vi "Prepare DCPower.vi"(8 "error in":errorcluster, 9 "Channel List in":string, 10 "Instrument Handle in":refnum<k15> caption="instrument handle", 11 "Measurement Configuration in":T1={"Resource Name"="", "Measure Trigger Source"="", "Run Until"=6.0, "Current Limit"=0.01, "Voltage Level"=0.01, "Current Limit Range"=0.0, "Voltage Level Range"=5.0, "Aperture Time"=0.01666, "Current Unit"="mA", "Delimited Text"=","} {"Aperture Time" format="%#_6ps"; "Voltage Level Range" format="%#_6pV"; "Current Limit Range" format="%#_6pA"; "Voltage Level" format="%#_6pV"; "Current Limit" format="%#_6pA"; "Run Until" min=1.0 step=1.0 format="%#_g Samples"}) -> (0 "error out":errorcluster, 1 "Channel List out":string, 2 "Instrument Handle out":refnum<k15>, 3 "Measurement Configuration out":T1 {"Aperture Time" format="%#_6ps"; "Voltage Level Range" format="%#_6pV"; "Current Limit Range" format="%#_6pA"; "Voltage Level" format="%#_6pV"; "Current Limit" format="%#_6pA"; "Run Until" min=1.0 step=1.0 format="%#_g Samples"})   [LabVIEW 2025, in "DCPower Single Meas Per Trigger.lvclass"]
uses:
  DCPower Single Meas Per Trigger.lvclass
  Measurement Configuration.ctl
  <instrlib>/niDCPower/nidcpower.llb/niDCPower Output Function.ctl
  <instrlib>/niDCPower/nidcpower.llb/niDCPower Auto Zero.ctl
  <instrlib>/niDCPower/nidcpower.llb/niDCPower Aperture Time Units.ctl
  DCPower Single Meas Per Trigger.lvclass/DCPower Single Meas Per Trigger.ctl
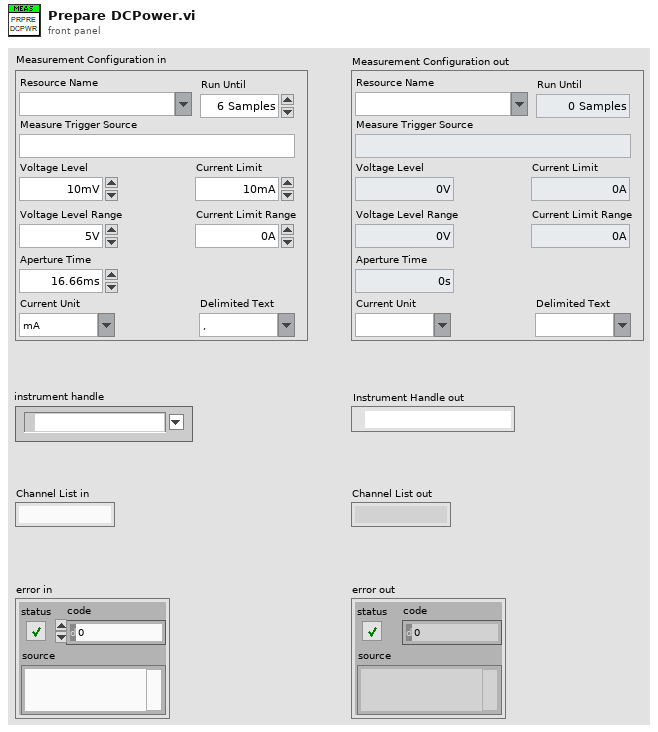
[diagram p1: front panel]
types:
  T1 = typedef "DCPower Single Meas Per Trigger.lvclass/Measurement Configuration.ctl" = cluster{"Resource Name":string, "Measure Trigger Source":string, "Run Until":dbl, "Current Limit":dbl, "Voltage Level":dbl, "Current Limit Range":dbl, "Voltage Level Range":dbl, "Aperture Time":dbl, "Current Unit":string, "Delimited Text":string}
  T2 = typedef "niDCPower Auto Zero.ctl" = i32
  T3 = typedef "niDCPower Output Function.ctl" = i32
  T4 = typedef "niDCPower Aperture Time Units.ctl" = i32
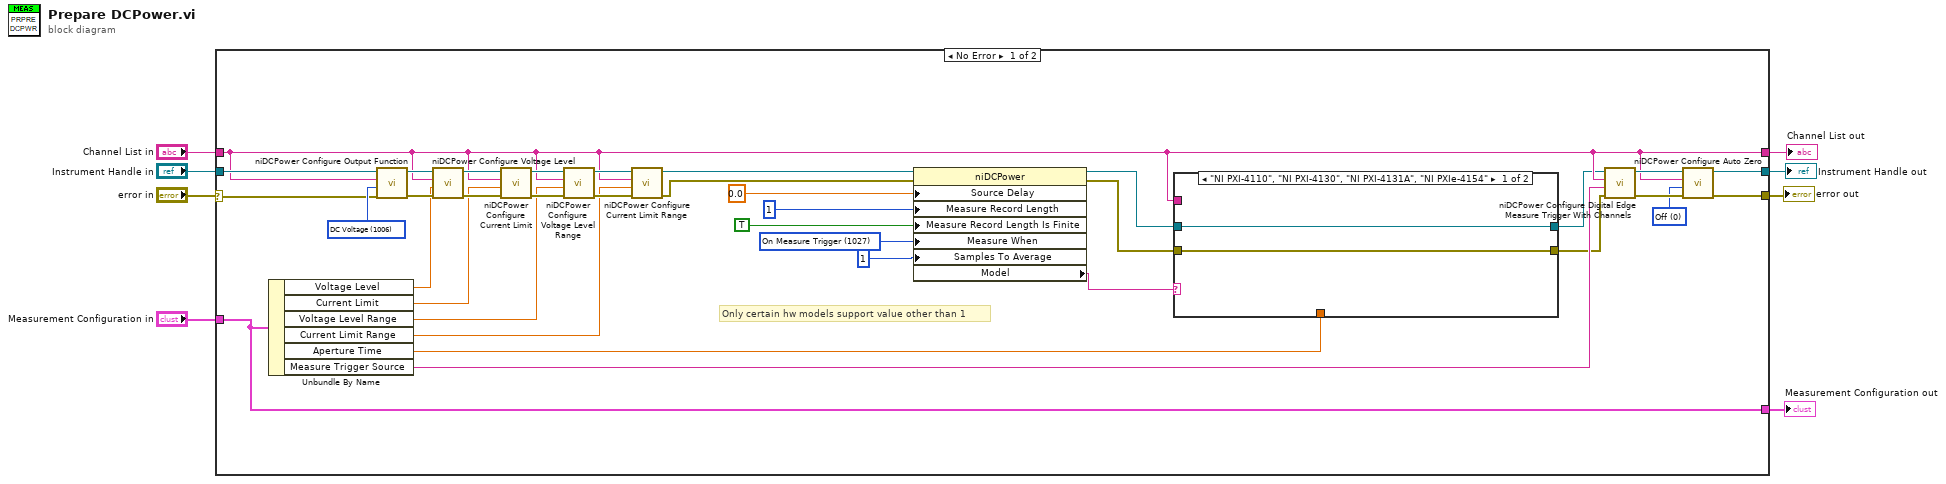
[diagram p0: block diagram]
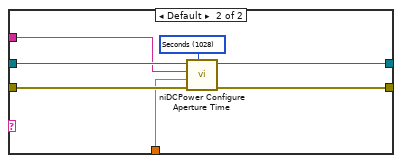
[diagram p2: hidden frame]
diagram:
  n1 = case shown="No Error" "error in" {
    selector: "error in" -> [w28 w56]
    tunnel: "Measurement Configuration in" -> [w26 w54]
    tunnel: [w19 w56] -> w7
    tunnel: "Instrument Handle in" -> [w29 w57]
    tunnel: [w17 w57] -> w5
    tunnel: "Channel List in" -> [w15 w55]
    tunnel: [w15 w55] -> w2
    tunnel: [w26 w54] -> w1
    frame No Error {
      w16 = T2 0 items=["Off"=0, "Once"=1024, "On"=1] ("auto zero")
      w23 = 1027 items=["Automatically after Source Complete"=1025, "On Demand"=1026, "On Measure Trigger"=1027] ("Measurement:Advanced:Measure When")
      w34 = T3 1006 items=["DC Voltage"=1006, "DC Current"=1007, "Pulse Voltage"=1049, "Pulse Current"=1050] ("output function")
      # "Only certain hw models support value other than 1"
      n2 = Unbundle By Name(w26) -> ("Voltage Level"=w33:dbl, "Current Limit"=w32:dbl, "Voltage Level Range"=w31:dbl, "Current Limit Range"=w30:dbl, "Aperture Time"=w10:dbl, "Measure Trigger Source"=w20:string)
      n3 = call <instrlib>:"niDCPower Configure Output Function.vi"("error in (no error)"=w28, "output function"=w34, "channel name"=w15, "instrument handle"=w29) -> ("error out"=w35:errorcluster, "instrument handle out"=w36:refnum<k15>)  [unwired: 6 out]
      n4 = call <instrlib>:"niDCPower Configure Voltage Level.vi"("error in (no error)"=w35, "voltage level"=w33, "channel name"=w15, "instrument handle"=w36) -> ("error out"=w43:errorcluster, "instrument handle out"=w44:refnum<k15>)  [unwired: 6 out]
      n5 = call <instrlib>:"niDCPower Configure Current Limit.vi"("error in (no error)"=w43, "current limit"=w32, "channel name"=w15, "instrument handle"=w44) -> ("error out"=w42:errorcluster, "instrument handle out"=w41:refnum<k15>)  [unwired: 1 in, 5 out]
      n6 = call <instrlib>:"niDCPower Configure Voltage Level Range.vi"("error in (no error)"=w42, "voltage level range"=w31, "channel name"=w15, "instrument handle"=w41) -> ("error out"=w40:errorcluster, "instrument handle out"=w39:refnum<k15>)  [unwired: 6 out]
      n7 = call <instrlib>:"niDCPower Configure Current Limit Range.vi"("error in (no error)"=w40, "current limit range"=w30, "channel name"=w15, "instrument handle"=w39) -> ("error out"=w37:errorcluster, "instrument handle out"=w38:refnum<k15>)  [unwired: 6 out]
      n8 = property class="niDCPower"(reference=w38, error in=w37, "Source Delay"=0.0 ("Source:Advanced:Source Delay"), "Measure Record Length"=1 ("Measurement:Measure Record Length"), "Measure Record Length Is Finite"=TRUE ("Measurement:Measure Record Length Is Finite"), "Measure When"=w23, "Samples To Average"=1 ("Measurement:Samples To Average")) -> (reference out=w14:refnum<k15>, error out=w13:errorcluster, "Model"=w9:string)
      n9 = case shown="\"NI PXI-4110\", \"NI PXI-4130\", \"NI PXI-4131A\", \"NI PXIe-4154\"" w9 {
        tunnel: w14 -> [w46 w53]
        tunnel: w13 -> [w45 w52]
        tunnel: [w45 w50] -> w11
        tunnel: [w46 w49] -> w12
        tunnel: w15 -> [_ w48]
        tunnel: w10 -> [_ w47]
        frame "NI PXI-4110", "NI PXI-4130", "NI PXI-4131A", "NI PXIe-4154" {
        }
        frame Default {
          w51 = T4 1028 items=["Seconds"=1028, "Powerline Cycles"=1029] ("aperture time units")
          n10 = call <instrlib>:"niDCPower Configure Aperture Time.vi"("aperture time units"=w51, "error in (no error)"=w52, "aperture time"=w47, "channel name"=w48, "instrument handle"=w53) -> ("error out"=w50:errorcluster, "instrument handle out"=w49:refnum<k15>)  [unwired: 5 out]
        }
      }
      n11 = call <instrlib>:"niDCPower Configure Digital Edge Measure Trigger With Channels.vi"("error in (no error)"=w11, "input terminal"=w20, "channel name"=w15, "instrument handle"=w12) -> ("error out"=w21:errorcluster, "instrument handle out"=w18:refnum<k15>)  [unwired: 6 in]
      n12 = call <instrlib>:"niDCPower Configure Auto Zero.vi"("error in (no error)"=w21, "auto zero"=w16, "channel name"=w15, "instrument handle"=w18) -> ("error out"=w19:errorcluster, "instrument handle out"=w17:refnum<k15>)  [unwired: 6 in]
    }
    frame Error {
    }
  }
  "error out" <- w7
  "Instrument Handle out" <- w5
  "Channel List out" <- w2
  "Measurement Configuration out" <- w1
